vi "Scan read v_2 axis (SubVI).vi"(6 "Y":i32, 7 "General VI":refnum<vi>, 8 "error in (no error)":errorcluster, 9 "Y_size":i32, 10 "X_size":i32, 11 "VISA Refnum in":refnum<visa-resource-name>) -> (0 "error out":errorcluster, 2 "value":dbl[](array[numeric]), 3 "VISA resource name out":refnum<visa-resource-name>)   [LabVIEW 2018]
uses:
  GlobalStop.vi
  <vilib>/regexp/Match Regular Expression.xnode
panel:
  out "X":i32
  out "succes, %":i32
  out "err":errorcluster
  out "ADC":i32[](array[numeric])
  out "str_array":string[][](array[string])
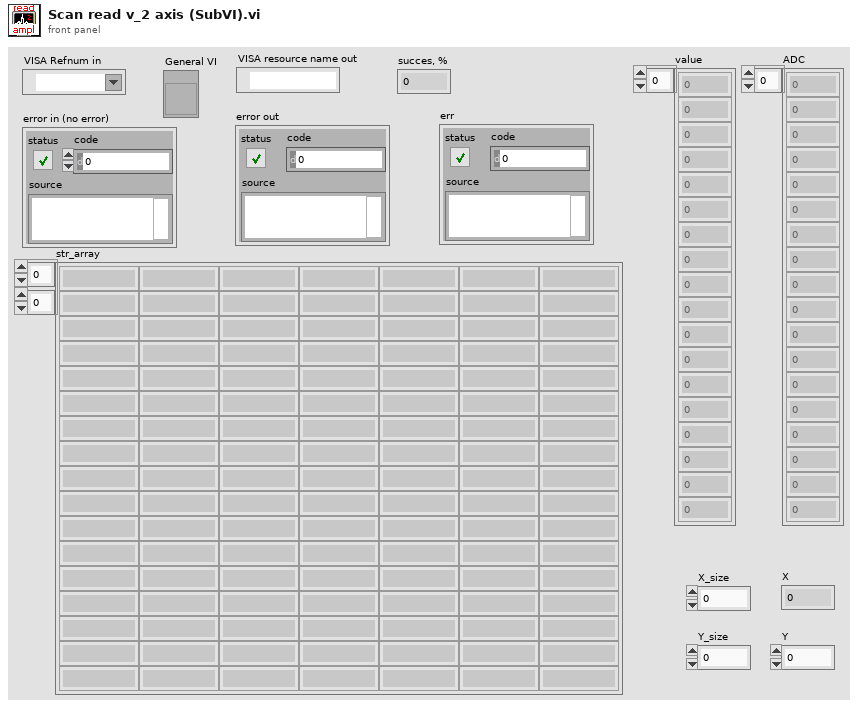
[diagram p1: front panel]
types:
  T1 = enum32{"Invalid", "Standard", "Closed", "Hidden", "Minimized", "Maximized"}
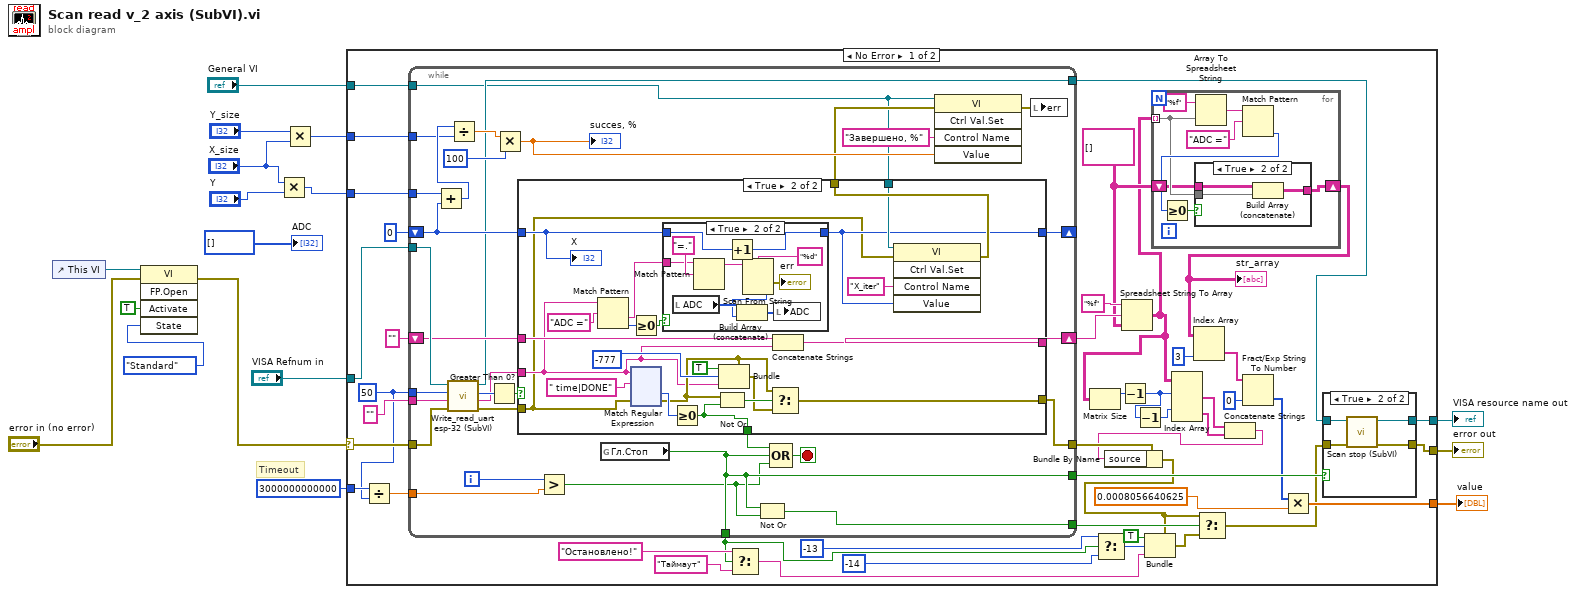
[diagram p0: block diagram]
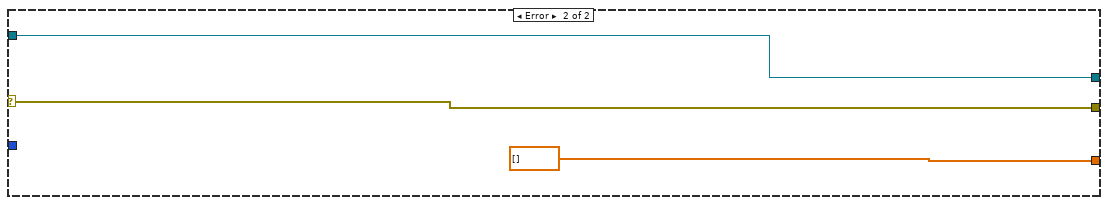
[diagram p6: hidden frame]
diagram:
  # "Timeout"
  n1 = control-ref of="This VI"() -> (w4:refnum<vi>)
  n2 = invoke class="VI" method="FP.Open"(reference=w4, error in="error in (no error)", "Activate"=TRUE, "State"=T1."Standard") -> (error out=w1:errorcluster)  [unwired: 1 in, 4 out]
  n3 = Multiply(x="X_size", y="Y") -> (x*y=w7:i32)
  n4 = Multiply(x="Y_size", y="X_size") -> (x*y=w8:i32)
  n5 = case shown="No Error" w1 {
    selector: w1 -> [w60 w264]
    tunnel: "VISA Refnum in" -> [w62 w265]
    tunnel: [w55 w265] -> w16
    tunnel: [w44 dbl[] []] -> w13
    tunnel: [w53 w264] -> w15
    tunnel: i64 3000000000000 -> [w50 _]
    tunnel: w8 -> [w30 _]
    tunnel: w7 -> [w29 _]
    tunnel: "General VI" -> [w28 _]
    frame No Error {
      w21 = string[][] [] ("Array")
      w49 = u32 50 ("milliseconds to wait")
      n6 = Divide(x=w50, y=w49) -> (x/y=w48:dbl)
      n7 = while {
        tunnel: w49 -> [w111]
        tunnel: "" ("write buffer") -> [w108]
        tunnel: [w97] -> w54
        tunnel: [w96] -> w24
        tunnel: [w96] -> w52
        tunnel: w48 -> [w102]
        shift-right: [w106] -> w43
        shift-left: "" -> [w105]
        tunnel: w62 -> [w110]
        shift-right: [w94] -> _
        shift-left: 0 -> [w91]
        tunnel: w30 -> [w89]
        tunnel: w29 -> [w88]
        tunnel: w28 -> [w81]
        tunnel: [w83] -> w22
        tunnel: w60 -> [w109]
        tunnel: [w86] -> w40
        i -> [w103]
        stop <- w104 stop-if-true
        n8 = Add(x=w88, y=w91) -> (x+y=w90:i32)
        n9 = call "Write_read_uart esp-32 (SubVI).vi"("error in (no error)"=w109, "write buffer"=w108, "milliseconds to wait"=w111, "VISA Refnum in"=w110) -> ("error out 4"=w100:errorcluster, "read buffer"=w98:string, "read bite"=w107:u32, "VISA resource name out"=w83:refnum<visa-resource-name>)
        n10 = Divide(x=w90, y=w89) -> (x/y=w93:dbl)
        n11 = Greater Than 0?(x=w107) -> (x > 0?=w99:bool)
        n12 = Multiply(x=w93, y=100) -> (x*y=w85:dbl)
        "succes, %" <- w85
        n13 = case shown="True" w99 {
          selector: w99 -> [w115 _]
          tunnel: [w114 w137] -> w106
          tunnel: w105 -> [w114 w136]
          tunnel: [w115 w128] -> w101
          tunnel: w98 -> [_ w127]
          tunnel: w100 -> [w112 w116]
          tunnel: [w112 w121] -> w86
          tunnel: w91 -> [w113 w122]
          tunnel: [w113 w117] -> w94
          tunnel: [w112 w120] -> w82
          tunnel: w81 -> [_ w119]
          frame False {
          }
          frame True {
            n14 = Match Pattern(string=w127, regular expression="ADC =") -> (after substring=w123:string, offset past match=w125:i32)  [unwired: 1 in, 2 out]
            n15 = Greater Or Equal To 0?(x=w125) -> (x >= 0?=w124:bool)
            n16 = xnode "Match Regular Expression"("input string"=w127, "regular expression"=" time|DONE", "error in"=w116) -> ("offset past match"=w134:i32, "error out"=w129:errorcluster)  [unwired: 3 in, 3 out]
            n17 = case shown="True" w124 {
              tunnel: w123 -> [_ w145]
              tunnel: w122 -> [w138 w140]
              tunnel: [w138 w139] -> w117
              frame False {
              }
              frame True {
                n18 = local read "ADC"() -> (w143:i32[])
                n19 = Match Pattern(string=w145, regular expression="=.") -> (before substring=w147:string)  [unwired: 1 in, 3 out]
                n20 = Increment(x=w140) -> (x+1=w139:i32)
                n21 = Scan From String(format string="%d", input string=w147) -> (error out=→"err":errorcluster, output 1=w142:i32)  [unwired: 3 in, 2 out]
                n22 = Build Array (concatenate)(w143, w142) -> (w141:i32[])
                n23 = local write "ADC"(w141) -> ()
              }
            }
            n24 = Greater Or Equal To 0?(x=w134) -> (x >= 0?=w128:bool)
            n25 = Not Or(1:w128, 2:w129) -> (0:w131:bool)
            n26 = Bundle(cluster=w129, "status"=TRUE, "code"=-777, "source"=w127) -> (w130:errorcluster)
            n27 = Select(t=w129, s=w131, f=w130) -> (s? t:f=w121:errorcluster)
            n28 = Concatenate Strings(w136, w127) -> (w137:string)
            n29 = invoke class="VI" method="Ctrl Val.Set"(reference=w119, error in=w116, "Control Name"="X_iter", "Value"=w117) -> (error out=w120:errorcluster)  [unwired: 1 in, 4 out]
            "X" <- w122
          }
        }
        n30 = Greater?(x=w103, y=w102) -> (0:w95:bool)
        n31 = global read "GlobalStop.vi" "Гл.Стоп"() -> (w96:bool)
        n32 = Not Or(1:w95, 2:w96) -> (0:w97:bool)
        n33 = Compound Arithmetic op=OR(w101, w96, w95) -> (w104:bool)
        n34 = invoke class="VI" method="Ctrl Val.Set"(reference=w81, error in=w82, "Control Name"="Завершено, %", "Value"=w85) -> (error out=w84:errorcluster)  [unwired: 1 in, 4 out]
        n35 = local write "err"(w84) -> ()
      }
      n36 = Select(t="Остановлено!" ("regular expression"), s=w24, f="Таймаут") -> (s? t:f=w27:string)
      n37 = Select(t=-13 ("code"), s=w24, f=-14 ("code")) -> (s? t:f=w25:i32)
      n38 = Spreadsheet String To Array(format string="%f", spreadsheet string=w43, array type (2D Dbl)=w21) -> (array=w20:string[][])  [unwired: 1 in]
      n39 = Matrix Size(0:w20) -> (1:w39:i32)  [unwired: 1 out]
      n40 = Decrement(x=w39) -> (x-1=w38:i32)
      n41 = Decrement(x=w38) -> (x-1=w37:i32)
      n42 = for {
        tunnel: w20 -> [w66] mode=indexing
        shift-right: [w65] -> w19
        shift-left: w21 -> [w64]
        n43 = Array To Spreadsheet String(array=w66, 3:"%f" ("format string")) -> (spreadsheet string=w70:string)  [unwired: 1 in]
        n44 = Match Pattern(string=w70, regular expression="ADC =") -> (offset past match=w68:i32)  [unwired: 1 in, 3 out]
        n45 = Greater Or Equal To 0?(x=w68) -> (x >= 0?=w67:bool)
        n46 = case shown="True" w67 {
          tunnel: w66 -> [_ w74]
          tunnel: [w71 w73] -> w65
          tunnel: w64 -> [w71 w72]
          frame False {
          }
          frame True {
            n47 = Build Array (concatenate)(w72, w74) -> (w73:string[][])
          }
        }
      }
      "str_array" <- w19
      n48 = Index Array(array=w20, index (row) #1=w38, index (row) #2=w37) -> (element #1=w36:string[], element #2=w35:string[])  [unwired: 2 in]
      n49 = Index Array(array=w19, index (col)=3 ("index (row)")) -> (element=w18:string[])  [unwired: 1 in]
      n50 = Concatenate Strings(w36, w35) -> (w34:string)
      n51 = Bundle By Name(cluster=w40, "source"=w34) -> (w33:errorcluster)
      n52 = Bundle(cluster=w33, "status"=TRUE, "code"=w25, "source"=w27) -> (w51:errorcluster)
      n53 = Select(t=w33, s=w54, f=w51) -> (s? t:f=w41:errorcluster)
      n54 = Fract/Exp String To Number(string=w18, default (0 dbl)=i16 0 ("default (0 DBL)")) -> (number=w45:i16[])  [unwired: 3 out]
      n55 = Multiply(x=w45, y=0.0008056640625) -> (x*y=w44:dbl[])
      n56 = case shown="True" w52 {
        tunnel: w22 -> [w75 w80]
        tunnel: [w75 w79] -> w55
        tunnel: w41 -> [w76 w78]
        tunnel: [w76 w77] -> w53
        frame False {
        }
        frame True {
          n57 = call "Scan stop (SubVI).vi"("error in"=w78, "VISA Refnum in"=w80) -> ("error out"=w77:errorcluster, "VISA Refnum out"=w79:refnum<visa-resource-name>)  [unwired: 8 in]
        }
      }
    }
    frame Error {
    }
  }
  "error out" <- w15
  "VISA resource name out" <- w16
  "value" <- w13
  "ADC" <- i32[] [] ("POS")
